vi "Main Page.vi"(8 "error in (no error)":errorcluster, 11 "Node Ptr":T1 format="%.0x") -> (0 "error out":errorcluster)   [LabVIEW 2020, in "gRPC Data Server System Explorer.lvlib"]
uses:
  gRPC Data Server System Explorer.lvlib
  <vilib>/NI VeriStand/Custom Device API/Custom Device Item Ref.ctl
  <vilib>/NI VeriStand/Custom Device API/Custom Device API.lvlib
  Shared/gRPC Data Server Shared.lvlib
panel:
  in  "Async?":bool
  in  "Server Address":string
  in  "Server Certificate File (.crt)":path
  in  "Server Key File (.key)":path
  out "Version":string
  in  "SHDocVw.IWebBrowser":refnum<k7>(container)
  in  "Specific Header":cluster{"Section Name":string}={"Section Name"="gRPC Server Settings"}
  in  "General Header":cluster{"Section Name":string}={"Section Name"="General Custom Device Settings"}
  in  "Description":string
  in  "Name":string
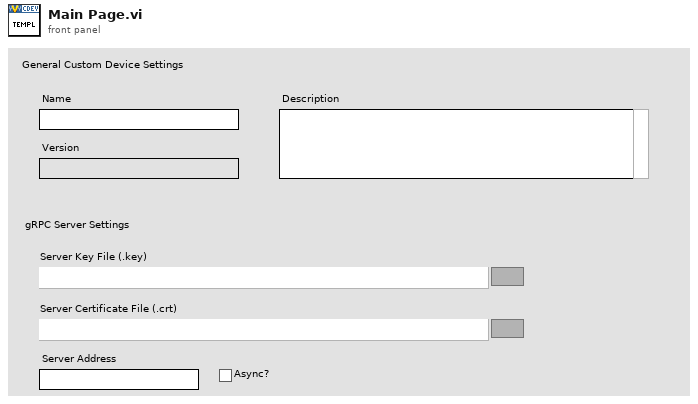
[diagram p1: front panel]
types:
  T1 = typedef "Custom Device API.lvlib/Custom Device Item Ref.ctl" = u64
  T2 = typedef "Custom Device API.lvlib/Custom Device Item Info.ctl" = cluster{"Name":string, "Is Channel":bool, "GUID":string, "Is Waveform":bool}
  T3 = typedef "gRPC Data Server Shared.lvlib/Compiled.Settings.ctl" = cluster{"Name":string, "Server Address":string, "Async?":bool, "Key File":path, "Cert File":path, "Channel Name":string[], "Initial Value":string[]}
  T4 = typedef "Custom Device API.lvlib/Custom Device Commands.ctl" = enum16{"Default", "Item renamed", "Shutdown", "Dynamic button pressed"}
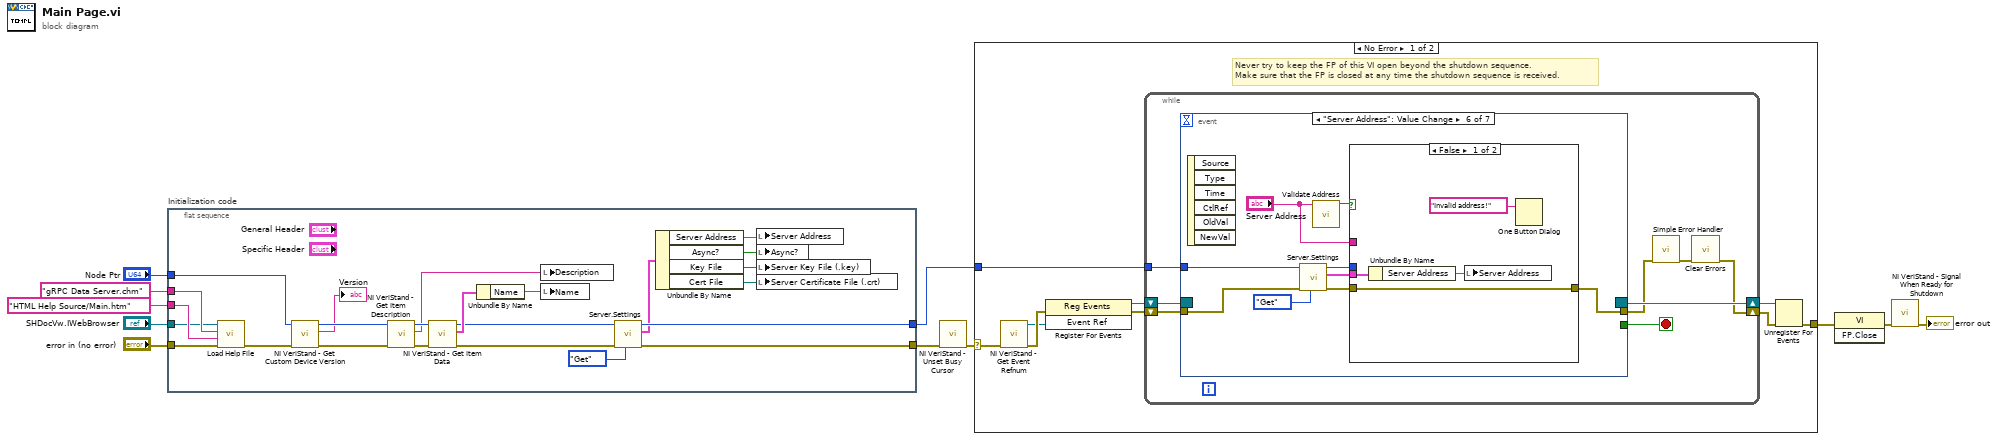
[diagram p0: block diagram]
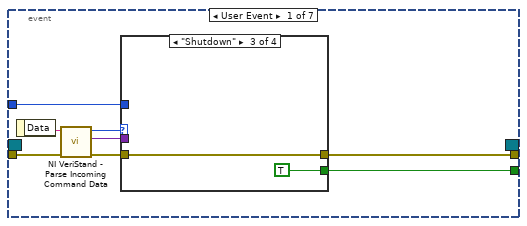
[diagram p2: hidden frame]
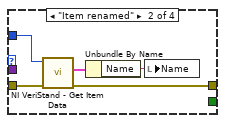
[diagram p4: hidden frame]
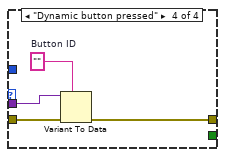
[diagram p5: hidden frame]
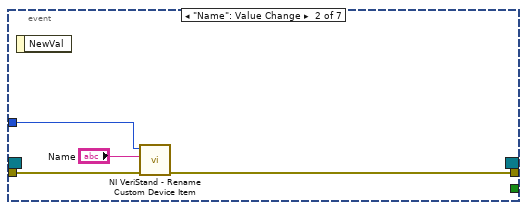
[diagram p6: hidden frame]
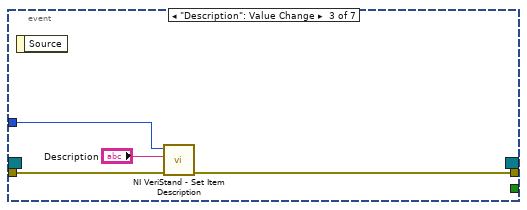
[diagram p7: hidden frame]
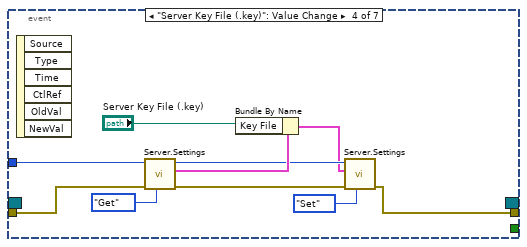
[diagram p8: hidden frame]
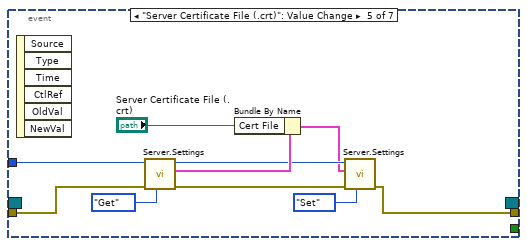
[diagram p9: hidden frame]
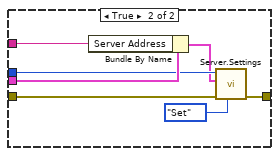
[diagram p10: hidden frame]
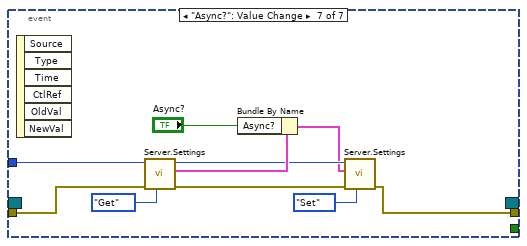
[diagram p11: hidden frame]
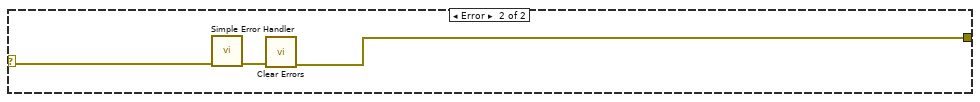
[diagram p12: hidden frame]
diagram:
  n1 = flat-sequence "Initialization code" {
    tunnel: "error in (no error)" -> [w26]
    tunnel: "Node Ptr" -> [w32]
    tunnel: [w17] -> w7
    tunnel: [w20] -> w4
    tunnel: "SHDocVw.IWebBrowser" -> [w22]
    tunnel: "HTML Help Source/Main.htm" ("HTML File") -> [w23]
    tunnel: "gRPC Data Server.chm" ("CD_CHM_FileName") -> [w24]
    frame #0 {
      n2 = call "Load Help File.vi"("error in (no error)"=w26, "HTML File to Load"=w23, "Main CHM File"=w24, "Browser"=w22) -> ("error out"=w25:errorcluster)  [unwired: 7 in]
      n3 = call <vilib>:"NI VeriStand - Get Custom Device Version.vi"("error in (no error)"=w25, "Device Ref in"=w32) -> ("error out"=w31:errorcluster, "Value"=→"Version":string, "Device Ref out"=w30:T1)  [unwired: 7 in]
      n4 = call <vilib>:"NI VeriStand - Get Item Description.vi"("error in (no error)"=w31, "Item Ref in"=w30) -> ("error out"=w34:errorcluster, "Description"=w27:string, "Item Ref out"=w35:T1)  [unwired: 7 out]
      n5 = call <vilib>:"NI VeriStand - Get Item Data.vi"("error in (no error)"=w34, "Item Ref in"=w35) -> ("error out"=w19:errorcluster, "Item Info"=w33:T2, "Item Ref out"=w21:T1)  [unwired: 7 out]
      n6 = Unbundle By Name(w33) -> ("Name"=w28:string)
      n7 = local write "Description"(w27) -> ()
      n8 = local write "Name"(w28) -> ()
      n9 = call "Server.Settings.vi"("Action"=enum8{"Get", "Set"}."Get", "error in (no error)"=w19, "Parent Ref in"=w21) -> ("error out"=w17:errorcluster, "Client Settings Out"=w16:T3, "Item Ref out"=w20:T1)  [unwired: 6 in]
      n10 = Unbundle By Name(w16) -> ("Server Address"=w15:string, "Async?"=w14:bool, "Key File"=w13:path, "Cert File"=w12:path)
      n11 = local write "Server Address"(w15) -> ()
      n12 = local write "Async?"(w14) -> ()
      n13 = local write "Server Key File (.key)"(w13) -> ()
      n14 = local write "Server Certificate File (.crt)"(w12) -> ()
    }
  }
  n15 = call <vilib>:"NI VeriStand - Unset Busy Cursor.vi"("error in (no error)"=w7) -> ("error out"=w6:errorcluster)  [unwired: 10 out]
  n16 = case shown="No Error" w6 {
    selector: w6 -> [w36 w133]
    tunnel: [w41 w131] -> w11
    tunnel: w4 -> [w37 _]
    frame No Error {
      # "Never try to keep the FP of this VI open beyond the shutdown sequence.\nMake sure that the FP is closed at any time the shutdown sequence is received."
      n17 = call <vilib>:"NI VeriStand - Get Event Refnum.vi"("error in (no error)"=w36) -> ("error out"=w44:errorcluster, "Event Ref"=w40:refnum<user-event>)  [unwired: 9 out]
      n18 = register-events(error in=w44, w40) -> (reference out=w38:refnum<event-registration>, error out=w39:errorcluster)  [unwired: 1 in]
      n19 = while {
        tunnel: w37 -> [w48]
        shift-right: [w45] -> w42
        shift-left: w39 -> [w51]
        shift-right: [w52] -> w43
        shift-left: w38 -> [w50]
        stop <- w49 stop-if-true
        n20 = event shown="[5] \"Server Address\": Value Change" {
          selector: w50 -> [_ _ _ _ _ _ _]
          dyn-events: [_ _ _ _ _ _ _] -> w52
          timeout: _ -> [_ _ _ _ _ _ _]
          tunnel: w51 -> [w60 w76 w79 w88 w98 w107 w128]
          tunnel: [w56 _ _ _ _ _ _] -> w49
          tunnel: [w55 w75 w78 w82 w93 w103 w123] -> w47
          tunnel: w48 -> [w54 w74 w80 w89 w99 w108 w129]
          event User Event {
            n21 = event-data() -> ("Data"=w59:string)  [unwired: 1 out]
            n22 = call <vilib>:"NI VeriStand - Parse Incoming Command Data.vi"("error in (no error)"=w60, "Incoming data"=w59) -> ("error out"=w58:errorcluster, "Outgoing data"=w53:variant, "Action"=w57:T4)  [unwired: 7 out]
            n23 = case shown="\"Shutdown\"" w57 {
              tunnel: w58 -> [w61 w66 w67 w72]
              tunnel: [_ _ TRUE _] -> w56
              tunnel: [w61 w63 w67 w69] -> w55
              tunnel: w54 -> [_ w65 _ _]
              tunnel: w53 -> [_ _ _ w71]
              frame "Default", Default {
              }
              frame "Item renamed" {
                n24 = call <vilib>:"NI VeriStand - Get Item Data.vi"("error in (no error)"=w66, "Item Ref in"=w65) -> ("error out"=w63:errorcluster, "Item Info"=w64:T2)  [unwired: 8 out]
                n25 = Unbundle By Name(w64) -> ("Name"=w62:string)
                n26 = local write "Name"(w62) -> ()
              }
              frame "Shutdown" {
              }
              frame "Dynamic button pressed" {
                w70 = ""  # Button ID
                n27 = Variant To Data(error in=w72, type=w70, Variant=w71) -> (error out=w69:errorcluster)  [unwired: 1 out]
              }
            }
          }
          event "Name": Value Change {
            n28 = event-data() -> ()  [unwired: 2 out]
            n29 = call <vilib>:"NI VeriStand - Rename Custom Device Item.vi"("error in (no error)"=w76, "New Name"="Name", "Item Ref in"=w74) -> ("error out"=w75:errorcluster)  [unwired: 1 in, 7 out]
          }
          event "Description": Value Change {
            n30 = event-data() -> ()  [unwired: 2 out]
            n31 = call <vilib>:"NI VeriStand - Set Item Description.vi"("error in (no error)"=w79, "Description"="Description", "Item Ref in"=w80) -> ("error out"=w78:errorcluster)  [unwired: 8 out]
          }
          event "Server Key File (.key)": Value Change {
            n32 = event-data() -> ()  [unwired: 7 out]
            n33 = call "Server.Settings.vi"("Action"=enum8{"Get", "Set"}."Get", "error in (no error)"=w88, "Parent Ref in"=w89) -> ("error out"=w85:errorcluster, "Client Settings Out"=w87:T3, "Item Ref out"=w86:T1)  [unwired: 6 in]
            n34 = Bundle By Name(cluster=w87, "Key File"="Server Key File (.key)") -> (w83:T3)
            n35 = call "Server.Settings.vi"("Action"=enum8{"Get", "Set"}."Set", "error in (no error)"=w85, "Client Settings In"=w83, "Parent Ref in"=w86) -> ("error out"=w82:errorcluster)  [unwired: 5 in, 2 out]
          }
          event "Server Certificate File (.crt)": Value Change {
            n36 = event-data() -> ()  [unwired: 7 out]
            n37 = call "Server.Settings.vi"("Action"=enum8{"Get", "Set"}."Get", "error in (no error)"=w98, "Parent Ref in"=w99) -> ("error out"=w95:errorcluster, "Client Settings Out"=w97:T3, "Item Ref out"=w96:T1)  [unwired: 6 in]
            n38 = Bundle By Name(cluster=w97, "Cert File"="Server Certificate File (.crt)") -> (w94:T3)
            n39 = call "Server.Settings.vi"("Action"=enum8{"Get", "Set"}."Set", "error in (no error)"=w95, "Client Settings In"=w94, "Parent Ref in"=w96) -> ("error out"=w93:errorcluster)  [unwired: 5 in, 2 out]
          }
          event "Server Address": Value Change {
            n40 = event-data() -> ()  [unwired: 7 out]
            n41 = call "Server.Settings.vi"("Action"=enum8{"Get", "Set"}."Get", "error in (no error)"=w107, "Parent Ref in"=w108) -> ("error out"=w104:errorcluster, "Client Settings Out"=w106:T3, "Item Ref out"=w105:T1)  [unwired: 6 in]
            n42 = call "Validate Address.vi"("IP Address"="Server Address") -> ("Valid"=w102:bool)  [unwired: 10 in]
            n43 = case shown="False" w102 {
              tunnel: w106 -> [w112 w120]
              tunnel: w105 -> [_ w119]
              tunnel: w104 -> [w111 w118]
              tunnel: [w111 w116] -> w103
              tunnel: "Server Address" -> [_ w114]
              frame False {
                n44 = Unbundle By Name(w112) -> ("Server Address"=w110:string)
                n45 = local write "Server Address"(w110) -> ()
                n46 = One Button Dialog(message="Invalid address!") -> ()  [unwired: 1 in, 1 out]
              }
              frame True {
                n47 = Bundle By Name(cluster=w120, "Server Address"=w114) -> (w117:T3)
                n48 = call "Server.Settings.vi"("Action"=enum8{"Get", "Set"}."Set", "error in (no error)"=w118, "Client Settings In"=w117, "Parent Ref in"=w119) -> ("error out"=w116:errorcluster)  [unwired: 5 in, 2 out]
              }
            }
          }
          event "Async?": Value Change {
            n49 = event-data() -> ()  [unwired: 7 out]
            n50 = call "Server.Settings.vi"("Action"=enum8{"Get", "Set"}."Get", "error in (no error)"=w128, "Parent Ref in"=w129) -> ("error out"=w125:errorcluster, "Client Settings Out"=w127:T3, "Item Ref out"=w126:T1)  [unwired: 6 in]
            n51 = Bundle By Name(cluster=w127, "Async?"="Async?") -> (w124:T3)
            n52 = call "Server.Settings.vi"("Action"=enum8{"Get", "Set"}."Set", "error in (no error)"=w125, "Client Settings In"=w124, "Parent Ref in"=w126) -> ("error out"=w123:errorcluster)  [unwired: 5 in, 2 out]
          }
        }
        n53 = call <vilib>:"Simple Error Handler.vi"("error in (no error)"=w47) -> ("error out"=w46:errorcluster)  [unwired: 1 in, 7 out]
        n54 = call <vilib>:"Clear Errors.vi"("error in (no error)"=w46) -> ("error out"=w45:errorcluster)  [unwired: 1 in, 5 out]
      }
      n55 = Unregister For Events(event registration refnum=w43, error in=w42) -> (error out=w41:errorcluster)
    }
    frame Error {
      n56 = call <vilib>:"Simple Error Handler.vi"("error in (no error)"=w133) -> ("error out"=w132:errorcluster)  [unwired: 1 in, 7 out]
      n57 = call <vilib>:"Clear Errors.vi"("error in (no error)"=w132) -> ("error out"=w131:errorcluster)  [unwired: 1 in, 5 out]
    }
  }
  n58 = invoke class="VI" method="FP.Close"(error in=w11) -> (error out=w10:errorcluster)  [unwired: 2 in, 2 out]
  n59 = call <vilib>:"NI VeriStand - Signal When Ready for Shutdown.vi"("error in (no error)"=w10) -> ("error out"=→"error out":errorcluster)  [unwired: 10 out]
